vi "Add Connection Callback.vi"(7 "Owner":refnum<class>, 8 "error in (no error)":errorcluster, 10 "Callback":refnum<vi>, 11 "Manager in":refnum<class "Manager.lvclass">) -> (0 "error out":errorcluster, 3 "Manager out":refnum<class "Manager.lvclass">)   [LabVIEW 2020, in "Stream-Simple-Msg.lvlib" / "Manager.lvclass"]
doc: "Registers a VI Callback reference to use when a new endpoint connects and is managed by this manager. A single VI callback can be used for both connections and disconnections as the state of the endpoint is passed in with the VI call.\n\nConnection callbacks are useful for sending initial state, identification, or configuration requests to newly connected systems and allowing software to implement auth mechanisms applied when endpoints connect. Likewise, handling disconnects to cleanup resources representing a connected endpoint is also useful."
uses:
  Manager.lvclass
  Endpoint/Endpoint.lvclass
  State Callback.ctl
  Manager.lvclass/Manager.ctl
  <vilib>/Utility/error.llb/Error Cluster From Error Code.vi
  <vilib>/ErrorRing/Error Ring.xnode
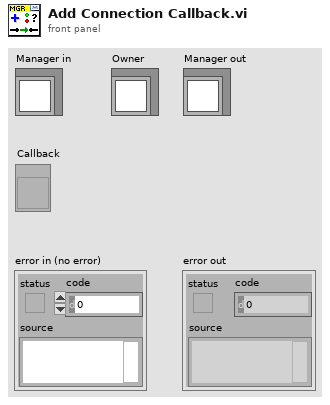
[diagram p1: front panel]
types:
  T1 = typedef "Stream-Simple-Msg.lvlib/Manager.lvclass/State Callback.ctl" = cluster{"Owner":refnum<class>, "VI":refnum<vi>, "Context":variant}
  T2 = typedef "Stream-Simple-Msg.lvlib/Manager.lvclass/Ref Data.ctl" = cluster{"Message Callbacks":map{string, T3[]}, "Endpoints":map{string, T4}, "Stream Endpoints":refnum<class "Endpoint.lvclass">[], "State Callbacks":T1[], "Stream Formats":T5[]}
  T3 = typedef "Stream-Simple-Msg.lvlib/Manager.lvclass/Callback.ctl" = cluster{"VI":refnum<vi>, "Owner":refnum<class>}
  T4 = typedef "Stream-Simple-Msg.lvlib/Manager.lvclass/Mapped Endpoint.ctl" = cluster{"Msg Endpoint":refnum<class "Endpoint.lvclass">, "Format":T5}
  T5 = typedef "Stream-Simple-Msg.lvlib/Format.ctl" = enum16{"LabVIEW Binary", "JSON"}
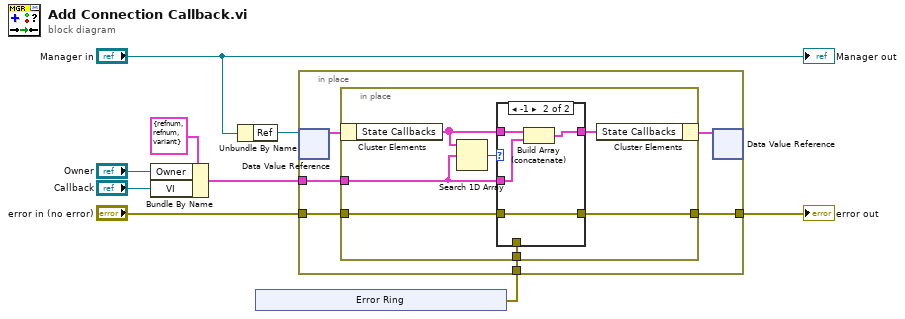
[diagram p0: block diagram]
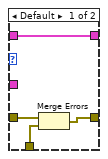
[diagram p2: hidden frame]
diagram:
  n1 = Bundle By Name(cluster=T1 {"Owner"=refnum, "VI"=refnum, "Context"=variant} ("State Callback"), "Owner"="Owner", "VI"="Callback") -> (w8:T1)
  n2 = Unbundle By Name("Manager in") -> ("Ref"=w9:refnum<data-value>)
  n3 = xnode "Error Ring"() -> ("error out"=w7:errorcluster)
  n4 = in-place {
    in-place-border: w8 -> [w13]
    in-place-border: "error in (no error)" -> [w12]
    in-place-border: w7 -> [w11]
    in-place-border: [w10] -> w2
    n5 = in-place-dvr #1(w9) -> (w15:T2)  [unwired: 1 out]
    n6 = in-place {
      in-place-border: w13 -> [w20]
      in-place-border: w12 -> [w18]
      in-place-border: w11 -> [w17]
      in-place-border: [w16] -> w10
      n7 = in-place-cluster #2(w15) -> ("State Callbacks"=w21:T1[])
      n8 = Search 1D Array(1D array=w21, element=w20) -> (index of element=w22:i32)  [unwired: 1 in]
      n9 = case shown="-1" w22 {
        tunnel: w21 -> [w26 w30]
        tunnel: w20 -> [_ w29]
        tunnel: [w26 w28] -> w19
        tunnel: w18 -> [w25 w27]
        tunnel: w17 -> [w24 _]
        tunnel: [w23 w27] -> w16
        frame Default {
          n10 = Merge Errors(w25, w24) -> (w23:errorcluster)
        }
        frame -1 {
          n11 = Build Array (concatenate)(w30, w29) -> (w28:T1[])
        }
      }
      n12 = in-place-cluster #2("State Callbacks"=w19) -> (w14:T2)
    }
    n13 = in-place-dvr #1(w14) -> ()  [unwired: 2 out]
  }
  "error out" <- w2
  "Manager out" <- "Manager in"
